vi "Discovery Server Get Discovery Service Address.vi"() -> (8 "address":string="localhost:42000")   [LabVIEW 2020]
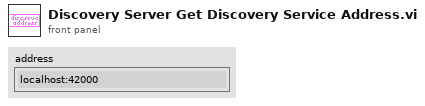
[diagram p1: front panel]
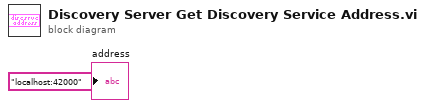
[diagram p0: block diagram]
diagram:
  "address" <- "localhost:42000" ("address")
